vi "init.vi"(8 "error in":errorcluster, 10 "TBM module configuration in":refnum<class "TBM module configuration.lvclass">, 11 "SQLite runtime in":refnum<class "SQLite runtime.lvclass">) -> (0 "error out":errorcluster, 1 "data allocations":T1, 2 "execution settings":T4, 3 "SQLite runtime out":refnum<class "SQLite runtime.lvclass">)   [LabVIEW 2014, in "SQLite runtime.lvclass"]
doc: "Provides an interface for initializing a module at runtime. While this interface performs no operations, a child should provide an override which may open any necessary references or sessions, allocate necessary memory, and perform any final configuration validataion before providing the full configuration <b>execution data</b> to the calling process."
uses:
  SQLite runtime.lvclass
  <vilib>/NI/Tag Bus Module Framework/module configuration/TBM module configuration.lvclass
  <vilib>/NI/Tag Bus Module Framework/runtime/execution settings.ctl
  <vilib>/NI/Tag Bus Module Framework/channel/data tables.ctl
  <vilib>/NI/Tag Bus/dictionary/data dictionary.lvclass
  <vilib>/NI/Tag Bus/dictionary table pair.ctl
  <vilib>/NI/Tag Bus/table/data table.ctl
  configuration/SQLite configuration.lvclass
  SQLite runtime.lvclass/SQLite runtime.ctl
  <vilib>/drjdpowell/SQLite Library/SQL Connection/Open (string).vi
  <vilib>/drjdpowell/SQLite Library/SQL Connection/Execute SQL (No results).vi
  <vilib>/drjdpowell/SQLite Library/SQL Connection/Connection.lvclass
  <vilib>/NI/Tag Bus Module Framework/channel/TBM channel.lvclass
  <vilib>/NI/Tag Bus Module Framework/runtime/TBM module execution interface.lvclass
  <vilib>/drjdpowell/SQLite Library/SQLite.lvlib
  <vilib>/NI/Tag Bus/tag bus.lvlib
  <vilib>/NI/Tag Bus/table/data table.lvlib
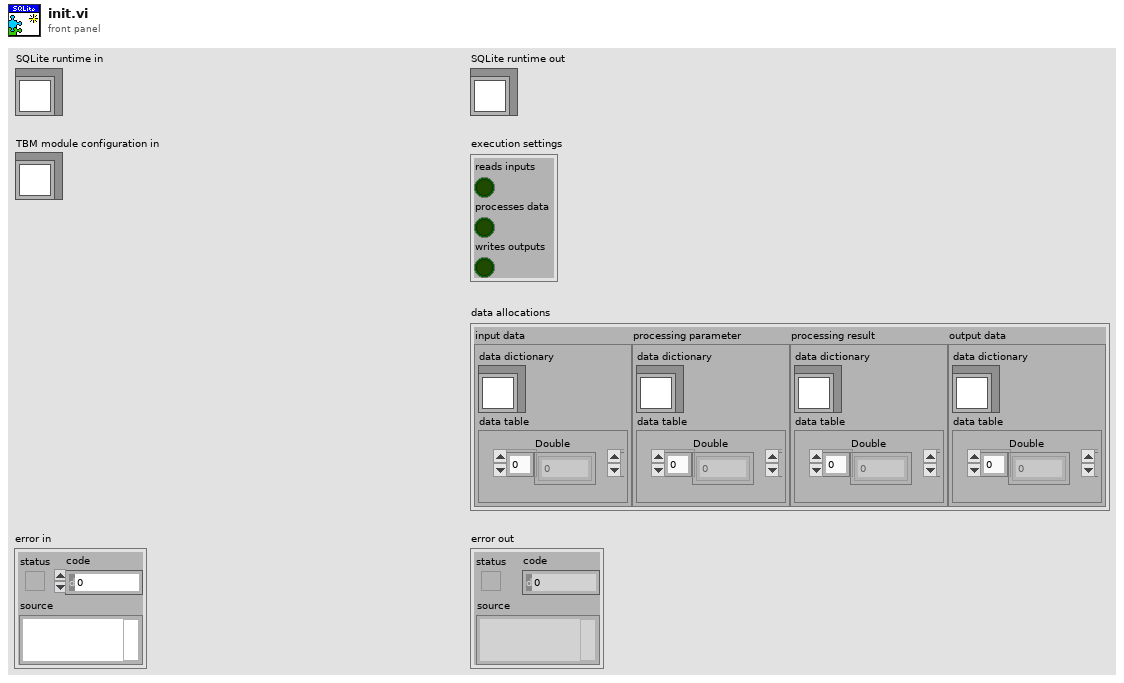
[diagram p1: front panel]
types:
  T1 = typedef "TBM channel.lvclass/data tables.ctl" = cluster{"input data":T2, "processing parameter":T2, "processing result":T2, "output data":T2}
  T2 = typedef "tag bus.lvlib/dictionary table pair.ctl" = cluster{"data dictionary":refnum<class "data dictionary.lvclass">, "data table":T3}
  T3 = typedef "tag bus.lvlib/data table.lvlib/data table.ctl" = cluster{"Double":dbl[], "Single":sgl[], "I64":i64[], "I32":i32[], "I16":i16[], "I8":i8[], "U64":u64[], "U32":u32[], "U16":u16[], "U8":u8[], "Boolean":bool[], "String":string[], "Array of Double":cluster{"DBL Array":dbl[]}[], "Array of Single":cluster{"SGL Array":sgl[]}[], "Array of I64":cluster{"I64 Array":i64[]}[], "Array of I32":cluster{"I32 Array":i32[]}[], "Array of I16":cluster{"I16 Array":i16[]}[], "Array of I8":cluster{"I8 Array":i8[]}[], "Array of U64":cluster{"U64 Array":u64[]}[], "Array of U32":cluster{"U32 Array":u32[]}[], "Array of U16":cluster{"U16 Array":u16[]}[], "Array of U8":cluster{"U8 Array":u8[]}[], "Array of Boolean":cluster{"Boolean Array":bool[]}[], "Array of String":cluster{"String Array":string[]}[]}
  T4 = typedef "TBM module execution interface.lvclass/execution settings.ctl" = cluster{"reads inputs":bool, "processes data":bool, "writes outputs":bool}
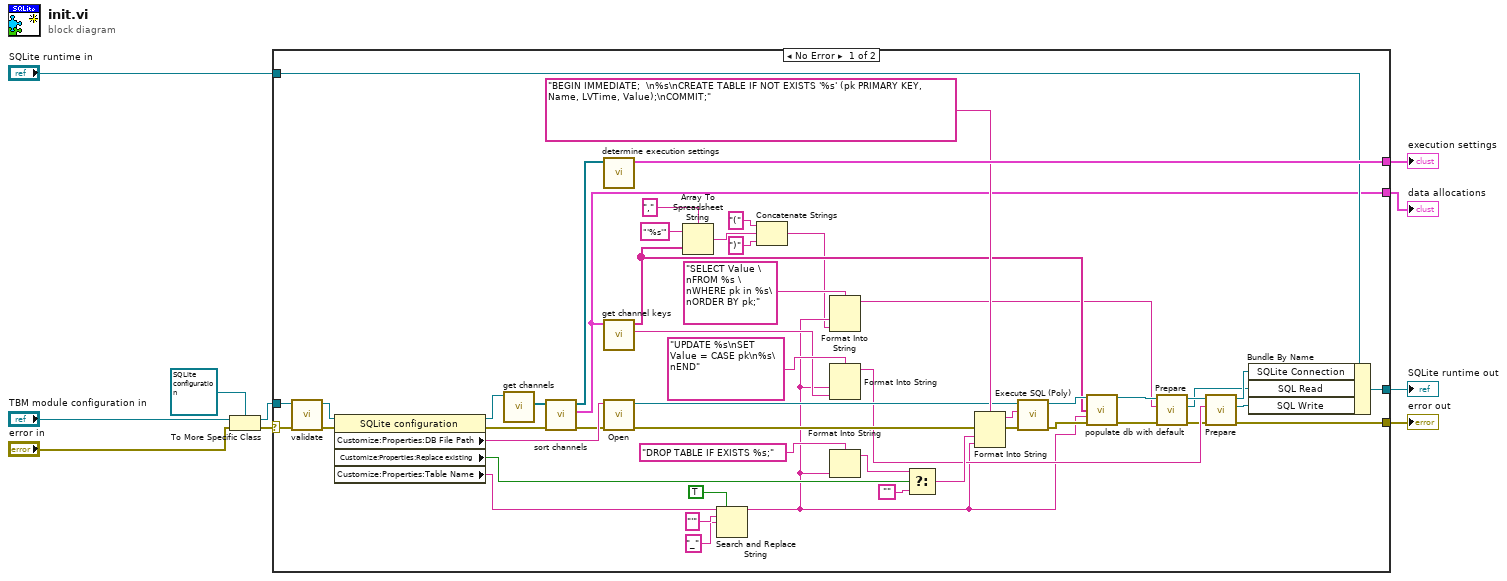
[diagram p0: block diagram]
diagram:
  n1 = To More Specific Class(target class=refnum<class "SQLite configuration.lvclass"> refnum ("Synchronous module configuration"), reference="TBM module configuration in", error in="error in") -> (specific class reference=w9:refnum<class "SQLite configuration.lvclass">, error out=w10:errorcluster)
  n2 = case shown="No Error" w10 {
    selector: w10 -> [w59 w62]
    tunnel: w9 -> [w58 _]
    tunnel: "SQLite runtime in" -> [w51 w63]
    tunnel: [w50 w63] -> w4
    tunnel: [w48 w62] -> w3
    tunnel: [w28 _] -> w1
    tunnel: [w61 _] -> w2
    frame No Error {
      n3 = call-dynamic "validate.vi"("error in"=w59, "SQLite configuration in"=w58) -> ("error out"=w55:errorcluster, "SQLite configuration out"=w56:refnum<class "SQLite configuration.lvclass">)  [unwired: 8 in]
      n4 = property class="SQLite configuration"(reference=w56, error in=w55) -> (reference out=w53:refnum<class "SQLite configuration.lvclass">, error out=w54:errorcluster, "Customize:Properties:DB File Path"=w52:string, "Customize:Properties:Replace existing"=w37:bool, "Customize:Properties:Table Name"=w36:string)
      n5 = call-dynamic "get channels.vi"("SQLite configuration in"=w53) -> ("channels"=w57:refnum<class "TBM channel.lvclass">[])  [unwired: 9 in, 1 out]
      n6 = call <vilib>:"sort channels.vi"("error in"=w54, "channels in"=w57) -> ("error out"=w49:errorcluster, "data allocations"=w28:T1, "channels out"=w60:refnum<class "TBM channel.lvclass">[])  [unwired: 7 in]
      n7 = call <vilib>:"determine execution settings.vi"("channels"=w60) -> ("execution settings"=w61:T4)  [unwired: 10 in]
      n8 = call "get channel keys.vi"("data allocations"=w28) -> ("output subquery"=w25:string, "input pk list"=w18:string[])  [unwired: 9 in]
      n9 = call-poly <vilib>:"Open.vi"("error in (no error)"=w49, "db file"=w52) -> ("error out"=w39:errorcluster, "SQLite Connection out"=w40:refnum<class "Connection.lvclass">)  [unwired: 8 in]
      n10 = Array To Spreadsheet String(delimiter (Tab)=",", array=w18, 3:"'%s'" ("format string")) -> (spreadsheet string=w17:string)
      n11 = Search and Replace String(replace all?=TRUE ("replace all? (F)"), input string=w36, search string="'", replace string="_" ("replace string (\"\")")) -> (result string=w13:string)  [unwired: 4 in, 3 out]
      n12 = Concatenate Strings("(" ("string"), w17, ")" ("string")) -> (w11:string)
      n13 = Format Into String(format string="SELECT Value \nFROM %s \nWHERE pk in %s\nORDER BY pk;" ("SQL"), w13, w11) -> (resulting string=w12:string)  [unwired: 2 in, 1 out]
      n14 = Format Into String(format string="UPDATE %s\nSET Value = CASE pk\n%s\nEND" ("SQL"), w13, w25) -> (resulting string=w29:string)  [unwired: 2 in, 1 out]
      n15 = Format Into String(format string="DROP TABLE IF EXISTS %s;" ("SQL"), w13) -> (resulting string=w32:string)  [unwired: 2 in, 1 out]
      n16 = Select(t=w32, s=w37, f="") -> (s? t:f=w43:string)
      n17 = Format Into String(format string="BEGIN IMMEDIATE;  \n%s\nCREATE TABLE IF NOT EXISTS '%s' (pk PRIMARY KEY, Name, LVTime, Value);\nCOMMIT;" ("SQL"), error in=w39, w43, w13) -> (resulting string=w41:string, error out=w38:errorcluster)  [unwired: 1 in]
      n18 = call-poly <vilib>:"Execute SQL (Poly).vi"("error in (no error)"=w38, "SQL"=w41, "SQLite Connection in"=w40) -> ("error out"=w22:errorcluster, "SQLite Connection out"=w24:refnum<class "Connection.lvclass">)  [unwired: 7 in]
      n19 = call "populate db with default.vi"("SQLite Connection in"=w24, "input pk list"=w18, "table name"=w13, "error in"=w22) -> ("SQLite Connection out"=w23:refnum<class "Connection.lvclass">, "error out"=w21:errorcluster)  [unwired: 10 in]
      n20 = call <vilib>:"Prepare.vi"("error in (no error)"=w21, "SQL"=w12, "SQLite Connection in"=w23) -> ("error out"=w26:errorcluster, "SQL Statement out"=w27:refnum<class "SQL Statement.lvclass">, "SQLite Connection out"=w45:refnum<class "Connection.lvclass">)  [unwired: 4 in, 2 out]
      n21 = call <vilib>:"Prepare.vi"("error in (no error)"=w26, "SQL"=w29, "SQLite Connection in"=w45) -> ("error out"=w48:errorcluster, "SQL Statement out"=w47:refnum<class "SQL Statement.lvclass">, "SQLite Connection out"=w46:refnum<class "Connection.lvclass">)  [unwired: 4 in, 2 out]
      n22 = Bundle By Name(cluster=w51, "SQLite Connection"=w46, "SQL Read"=w27, "SQL Write"=w47) -> (w50:refnum<class "SQLite runtime.lvclass">)
    }
    frame Error {
    }
  }
  "error out" <- w3
  "SQLite runtime out" <- w4
  "execution settings" <- w2
  "data allocations" <- w1
